vi "DSF.Engine.Memory.Buffer.Set Buffer Size.vi"(10 "buffer size":u64, 11 "Buffer in":refnum<class "DSF.Engine.Memory.Buffer.lvclass">) -> (3 "Buffer out":refnum<class "DSF.Engine.Memory.Buffer.lvclass">)   [LabVIEW 2017, in "DSF.Engine.lvlib" / "DSF.Engine.Memory.Buffer.lvclass"]
uses:
  DSF.Engine.Memory.Buffer.lvclass
  DSF.Engine.Memory.Buffer.lvclass/DSF.Engine.Memory.Buffer.ctl
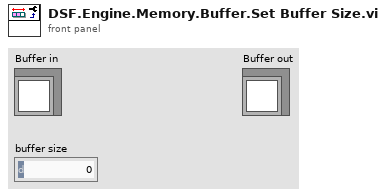
[diagram p1: front panel]
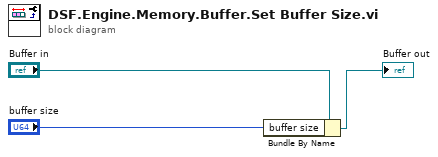
[diagram p0: block diagram]
diagram:
  n1 = Bundle By Name(cluster="Buffer in", "buffer size"="buffer size") -> (→"Buffer out":refnum<class "DSF.Engine.Memory.Buffer.lvclass">)
